vi "5024_Module_configure.vi"() -> ()   [LabVIEW 2010]
uses:
  ADAM Client/Sub VIs/ADAM Controls/Address.ctl
panel:
  in  "Output Range":u16(ring) items=["30   0 to 20mA", "31   4 to 20mA", "32   0 to 10V"]
  in  "Slew Rate":u16(ring) items=["Instant", "0.0625 V/sec", "0.125 V/sec", "0.250 V/sec", "0.500 V/sec", "1.000 V/sec", "2.000 V/sec", "4.000 V/sec", "8.000 V/sec", "16.000 V/sec", "32.000 V/sec", "64.000 V/sec"]
  in  "Address (all reqd.)":T1={"Main"=0, "Ch."=0, "Sub"=0, "Port Name"="MainNetwork"}
  in  "Data Format (ONLY ENG UNITS)":u16(ring) items=["Engineering Units", "% of FSR", "Hex", "Ohms (4013)"]
  out "Reply":string
  out "Message sent":string
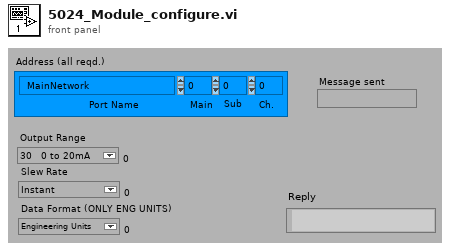
[diagram p1: front panel]
types:
  T1 = typedef "Address.ctl" = cluster{"Main":i32, "Ch.":i32, "Sub":i32, "Port Name":string}
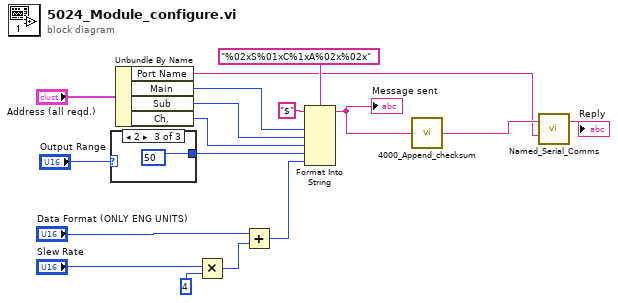
[diagram p0: block diagram]
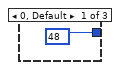
[diagram p2: hidden frame]
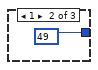
[diagram p3: hidden frame]
diagram:
  n1 = case shown="2" "Output Range" {
    tunnel: [48 49 50] -> w2
    frame 0, Default {
    }
    frame 1 {
    }
    frame 2 {
    }
  }
  n2 = Unbundle By Name("Address (all reqd.)") -> ("Port Name"=w1:string, "Main"=w9:i32, "Sub"=w10:i32, "Ch."=w11:i32)
  n3 = Multiply(x="Slew Rate", y=u16 4) -> (x*y=w7:u16)
  n4 = Add(x="Data Format (ONLY ENG UNITS)", y=w7) -> (x+y=w4:u16)
  n5 = Format Into String(format string="%02xS%01xC%1xA%02x%02x", initial string="$", w9, w10, w11, w2, w4) -> (resulting string=w15:string)  [unwired: 1 in, 1 out]
  "Message sent" <- w15
  n6 = call "4000_Append_checksum.vi"("ADAM command"=w15) -> ("ADAM string to send"=w13:string)
  n7 = call "Named_Serial_Comms.vi"("Write String"=w13, "Port Name"=w1) -> ("Read"=→"Reply":string)  [unwired: 10 in, 3 out]
